vi "drive test.vi"() -> ()   [LabVIEW 2009]
uses:
  DAQ enum.ctl
panel:
  out "CH3":dbl[](array[numeric]) format="%.2f"
  out "CH2":dbl[](array[numeric]) format="%.2f"
  out "CH1":dbl[](array[numeric]) format="%.2f"
  out "CH0":dbl[](array[numeric]) format="%.2f"
  in  "停止":bool
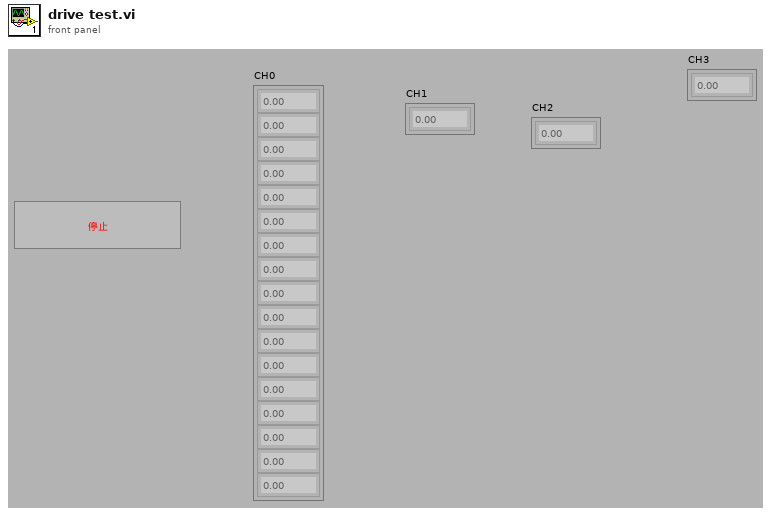
[diagram p1: front panel]
types:
  T1 = typedef "DAQ enum.ctl" = enum16{"open", "config", "start", "read", "stop", "noop", "close"}
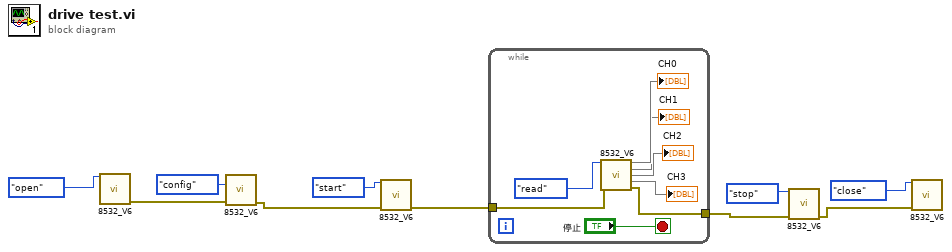
[diagram p0: block diagram]
diagram:
  n1 = call "8532_V6.vi"("enum"=DAQ_enum."open") -> ("错误输入（无错误） 2"=w5:errorcluster)  [unwired: 13 in, 1 out]
  n2 = call "8532_V6.vi"("enum"=DAQ_enum."config", "错误输入（无错误）"=w5) -> ("错误输入（无错误） 2"=w4:errorcluster)  [unwired: 12 in, 1 out]
  n3 = call "8532_V6.vi"("enum"=DAQ_enum."start", "错误输入（无错误）"=w4) -> ("错误输入（无错误） 2"=w3:errorcluster)  [unwired: 12 in, 1 out]
  n4 = while {
    tunnel: w3 -> [w16]
    tunnel: [w15] -> w2
    stop <- "停止" stop-if-true
    n5 = call "8532_V6.vi"("enum"=DAQ_enum."read", "错误输入（无错误）"=w16) -> (4:→"CH0", 6:→"CH1", 8:→"CH2", 10:→"CH3", "错误输入（无错误） 2"=w15:errorcluster)  [unwired: 8 in, 1 out]
  }
  n6 = call "8532_V6.vi"("enum"=DAQ_enum."stop", "错误输入（无错误）"=w2) -> ("错误输入（无错误） 2"=w1:errorcluster)  [unwired: 12 in, 1 out]
  n7 = call "8532_V6.vi"("enum"=DAQ_enum."close", "错误输入（无错误）"=w1) -> ()  [unwired: 12 in, 2 out]
